vi "DRAM FIFO (U256).vi"(0 "Input Data":T5, 1 "reset":bool, 2 "Memory":T6, 3 "arbiter configuration":T4={"write grant time (clocks)"=100, "read grant time (clocks)"=100}, 5 "fifo depth":T1=8 items=["4"=2, "8"=3, "16"=4, "32"=5, "64"=6, "128"=7, "256"=8, "512"=9, "1024"=10, "2048"=11, "4096"=12, "8192"=13, "16384"=14, "32768"=15, "65536"=16, "131072"=17, "262144"=18, "524288"=19, "1048576"=20, "2097152"=21, "4194304"=22, "8388608"=23, "16777216"=24, "33554432"=25, "67108864"=26, "134217728"=27, "268435456"=28, "536870912"=29, "1073741824"=30, "2147483648"=31, "4294967296"=32], 7 "Sim_DRAM Skew":fxp<+,32,0>, 11 "input valid":bool, 14 "ready for output":bool=TRUE) -> (4 "Output Data":T5, 6 "state":T7, 8 "bank0.data":T2, 10 "Bank1.data":T2, 12 "Ready for Input":bool, 15 "Output Valid":bool)   [LabVIEW 2012, in "FIFO.lvlib"]
doc: "This VI creates a wider datapath (U256) FIFO using two DRAM U128 FIFO's (RF-RIO).\nThe outputs of the two DRAM FIFO's are cascaded to enforce writes and reads without glitches.\n\n<b> To do: </b>\nTest cascade logic for next tick glitch\nTest throughput of the DRAM"
uses:
  <userlib>/FPGA Library/Code Development/DRAM/RF-RIO/FIFO/FIFO/FPGA/FIFO.lvlib
  <userlib>/FPGA Library/Code Development/DRAM/RF-RIO/FIFO/FIFO/FPGA/Public/FIFO State.ctl
  <userlib>/FPGA Library/Code Development/DRAM/2 Bank DRAM/Data Type (256).ctl
  <userlib>/FPGA Library/Code Development/DRAM/RF-RIO/Memory/1.0.0/FPGA/Public/Timeslot Arbiter Configuration.ctl
  <userlib>/FPGA Library/Code Development/DRAM/RF-RIO/Memory/1.0.0/FPGA/Public/Retrieve Data (128-Bit).ctl
  <userlib>/FPGA Library/Code Development/DRAM/RF-RIO/Memory/1.0.0/FPGA/Public/U128.ctl
  <userlib>/FPGA Library/Code Development/DRAM/RF-RIO/FIFO/FIFO/FPGA/Private/FIFO Depth - 32-bit Address.ctl
  <userlib>/FPGA Library/Code Development/DRAM/RF-RIO/Memory/1.0.0/FPGA/Public/Write Data (128-Bit).ctl
  <instrlib>/FlexRIO/Libraries/Memory/FPGA/Interface/Read Request.ctl
  <userlib>/FPGA Library/Code Development/DRAM/2 Bank DRAM/Controls/Individual Bank Status.ctl
  <userlib>/FPGA Library/Code Development/DRAM/2 Bank DRAM/Controls/Cascaded Bank Status.ctl
  <userlib>/FPGA Library/Code Development/DRAM/RF-RIO/Memory/1.0.0/FPGA/Private/Process (DRAM 128-Bit).vi
  <instrlib>/FlexRIO/Libraries/Memory/FPGA/Memory.lvlib
  <userlib>/FPGA Library/Code Development/DRAM/RF-RIO/Memory/1.0.0/FPGA/niRFRIO Memory 1.0.0 FPGA.lvlib
panel:
  out "ready for write":bool
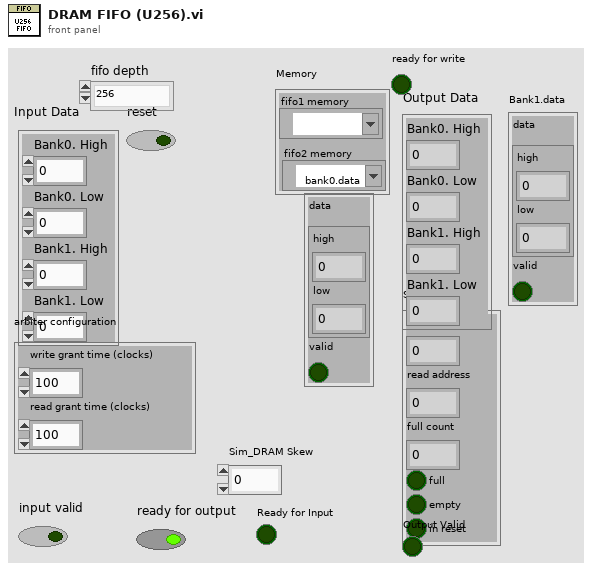
[diagram p1: front panel]
types:
  T1 = typedef "FIFO.lvlib/FIFO Depth - 32-bit Address.ctl" = u8
  T2 = typedef "FIFO.lvlib/niRFRIO Memory 1.0.0 FPGA.lvlib/Retrieve Data (128-Bit).ctl" = cluster{"data":T3, "valid":bool}
  T3 = typedef "FIFO.lvlib/niRFRIO Memory 1.0.0 FPGA.lvlib/U128.ctl" = cluster{"high":u64, "low":u64}
  T4 = typedef "FIFO.lvlib/niRFRIO Memory 1.0.0 FPGA.lvlib/Timeslot Arbiter Configuration.ctl" = cluster{"write grant time (clocks)":u16, "read grant time (clocks)":u16}
  T5 = typedef "Data Type (256).ctl" = cluster{"Bank0. High":u64, "Bank0. Low":u64, "Bank1. High":u64, "Bank1. Low":u64}
  T6 = cluster{"fifo1 memory":refnum<k21>, "fifo2 memory":refnum<k21>}
  T7 = typedef "FIFO.lvlib/FIFO State.ctl" = cluster{"write address":u32, "read address":u32, "full count":u32, "full":bool, "empty":bool, "in reset":bool}
  T8 = typedef "Cascaded Bank Status.ctl" = cluster{"Banks In Sync?":bool, "RetrieveData from Bank  0":bool, "RetrieveData from Bank  1":bool, "ready for read request":bool, "ready for write":bool}
  T9 = typedef "Individual Bank Status.ctl" = cluster{"ready for read request":bool, "ready for write":bool}
  T10 = typedef "Memory.lvlib/Read Request.ctl" = cluster{"address":u32, "valid":bool}
  T11 = typedef "FIFO.lvlib/niRFRIO Memory 1.0.0 FPGA.lvlib/Write Data (128-Bit).ctl" = cluster{"address":u32, "data":T3, "byte enables":u16, "valid":bool}
  T12 = typedef "FIFO.lvlib/FIFO State - 32-bit Address.ctl" = cluster{"write address":u32, "read address":u32, "full count":u32, "full":bool, "empty":bool}
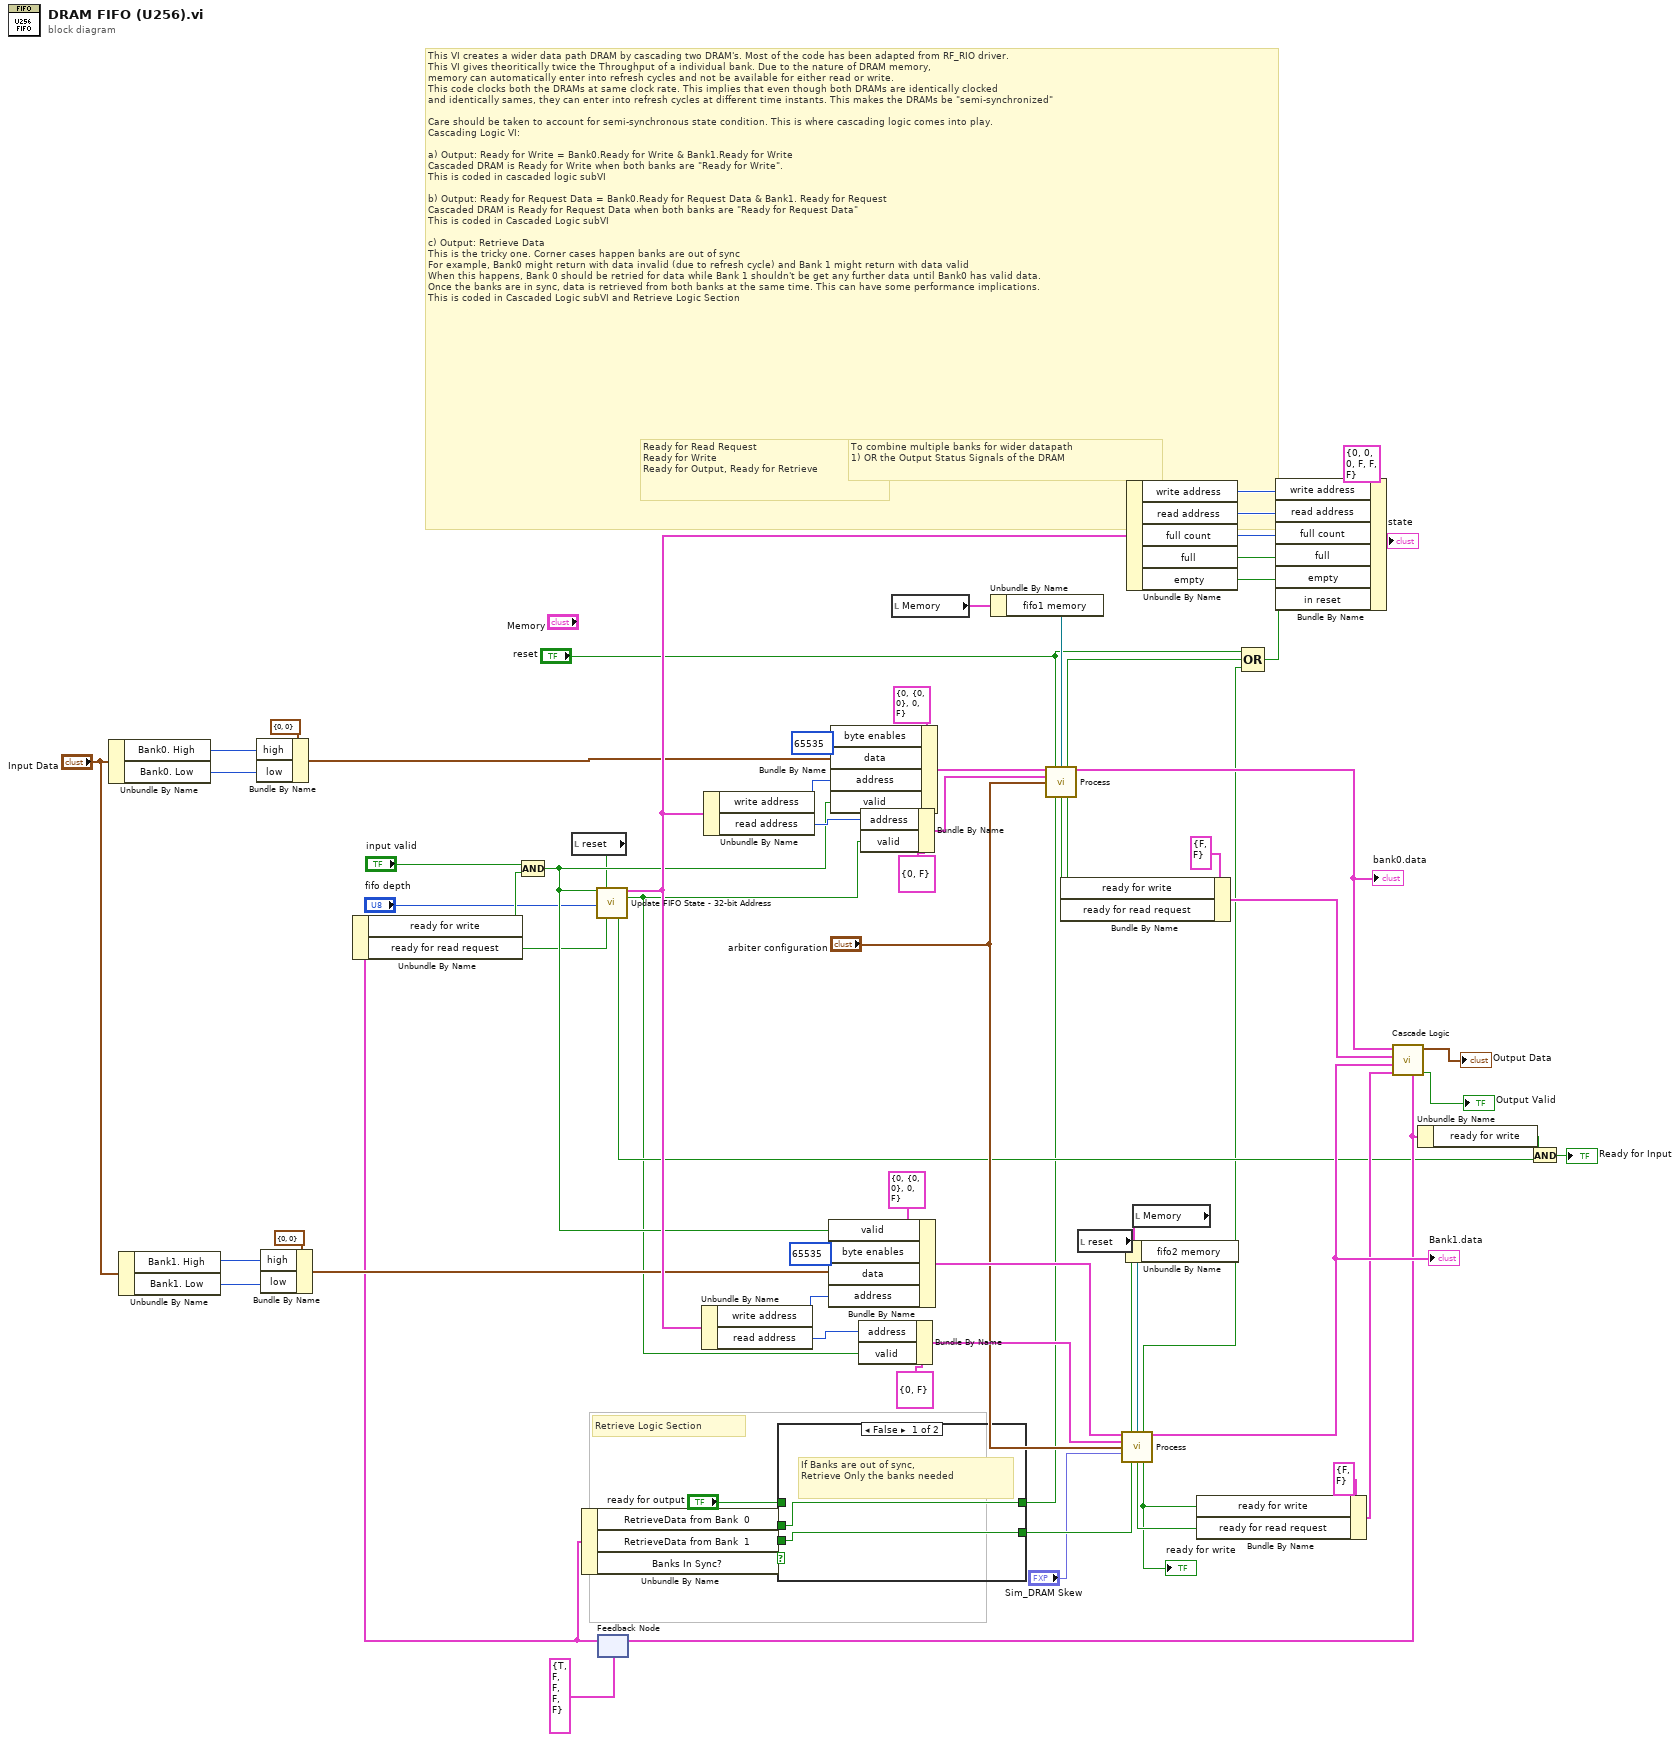
[diagram p0: block diagram]
diagram:
  # "Retrieve Logic Section"
  # "This VI creates a wider data path DRAM by cascading two DRAM's. Most of the code has been adapted from RF_RIO driver.\nThis VI gives theoritically twice the Throughput of a individual bank. Due to the nature of DRAM memory, \nmemory can automatically enter into refresh cycles and not be available for either read or write.\nThis code clocks both the DRAMs at same clock rate. This implies that even though both DRAMs are identically clocked\nand identically sames, they can enter into refresh cycles at different time instants. This makes the DRAMs be \"semi-synchronized\"\n\nCare should be taken to account for semi-synchronous state condition. This is where cascading logic comes into play.\nCascading Logic VI:\n\na) Output: Ready for Write = Bank0.Ready for Write & Bank1.Ready for Write\nCascaded DRAM is Ready for Write when both banks are \"Ready for Write\".\nThis is coded in cascaded logic subVI\n\nb) Output: Ready for Request Data = Bank0.Ready for Request Data & Bank1. Ready for Request\nCascaded DRAM is Ready for Request Data when both banks are \"Ready for Request Data\"\nThis is coded in Cascaded Logic subVI\n\nc) Output: Retrieve Data\nThis is the tricky one. Corner cases happen banks are out of sync\nFor example, Bank0 might return with data invalid (due to refresh cycle) and Bank 1 might return with data valid  \nWhen this happens, Bank 0 should be retried for data while Bank 1 shouldn't be get any further data until Bank0 has valid data.\nOnce the banks are in sync, data is retrieved from both banks at the same time. This can have some performance implications.\nThis is coded in Cascaded Logic subVI and Retrieve Logic Section"
  # "Ready for Read Request\nReady for Write\nReady for Output, Ready for Retrieve"
  # "To combine multiple banks for wider datapath\n1) OR the Output Status Signals of the DRAM"
  n1 = Unbundle By Name("Input Data") -> ("Bank0. High"=w48:u64, "Bank0. Low"=w47:u64)
  n2 = Unbundle By Name("Input Data") -> ("Bank1. High"=w43:u64, "Bank1. Low"=w42:u64)
  n3 = Bundle By Name(cluster=cluster{"high":u64, "low":u64} {"high"=0, "low"=0} ("input data"), "high"=w48, "low"=w47) -> (w46:cluster{"high":u64, "low":u64})
  n4 = Bundle By Name(cluster=cluster{"high":u64, "low":u64} {"high"=0, "low"=0} ("input data"), "high"=w43, "low"=w42) -> (w41:cluster{"high":u64, "low":u64})
  n5 = local read "reset"() -> (w17:bool)
  n6 = feedback #1(T8 {"Banks In Sync?"=TRUE, "RetrieveData from Bank  0"=FALSE, "RetrieveData from Bank  1"=FALSE, "ready for read request"=FALSE, "ready for write"=FALSE} ("Cascaded Bank Status")) -> (w21:T8)
  n7 = Unbundle By Name(w21) -> ("ready for write"=w26:bool, "ready for read request"=w1:bool)
  n8 = Compound Arithmetic op=AND("input valid", w26) -> (w33:bool)
  n9 = Unbundle By Name(w21) -> ("RetrieveData from Bank  0"=w8:bool, "RetrieveData from Bank  1"=w7:bool, "Banks In Sync?"=w22:bool)
  n10 = call <userlib>:"Update FIFO State - 32-bit Address.vi"("issue write"=w33, "reset"=w17, "fifo depth"="fifo depth", "ready for read request"=w1) -> ("state"=w52:T12, "issue read request"=w11:bool, "ready for write"=w19:bool)  [unwired: 9 in]
  n11 = Unbundle By Name(w52) -> ("write address"=w55:u32, "read address"=w57:u32)
  n12 = Unbundle By Name(w52) -> ("write address"=w70:u32, "read address"=w67:u32)
  n13 = case shown="False" w22 {
    tunnel: w8 -> [w75 _]
    tunnel: w7 -> [w74 _]
    tunnel: "ready for output" -> [_ w76]
    tunnel: [w75 w76] -> w5
    tunnel: [w74 w76] -> w4
    frame False {
      # "If Banks are out of sync,\nRetrieve Only the banks needed"
    }
    frame True {
      # "Retrieve Data = Ready for O/P"
      # "If banks are in sync, retriveve\ndata when ready for output is true"
    }
  }
  n14 = Bundle By Name(cluster=T11 {"address"=0, "data"={"high"=0, "low"=0}, "byte enables"=0, "valid"=FALSE} ("write data"), "valid"=w33, "byte enables"=u16 65535, "data"=w41, "address"=w55) -> (w51:T11)
  n15 = Bundle By Name(cluster=T11 {"address"=0, "data"={"high"=0, "low"=0}, "byte enables"=0, "valid"=FALSE} ("write data"), "byte enables"=u16 65535, "data"=w46, "address"=w70, "valid"=w33) -> (w71:T11)
  n16 = Bundle By Name(cluster=T10 {"address"=0, "valid"=FALSE} ("read request"), "address"=w57, "valid"=w11) -> (w50:T10)
  n17 = Bundle By Name(cluster=T10 {"address"=0, "valid"=FALSE} ("read request"), "address"=w67, "valid"=w11) -> (w68:T10)
  n18 = local read "Memory"() -> (w14:T6)
  n19 = Unbundle By Name(w14) -> ("fifo1 memory"=w39:refnum<k21>)
  n20 = call-poly <userlib>:"Process.vi"("write data"=w71, "reset"="reset", "memory"=w39, "read request"=w68, "arbiter configuration"="arbiter configuration", "ready for retrieve data (T)"=w5) -> ("in reset"=w58:bool, "retrieve data"=w36:T2, "ready for read request"=w28:bool, "ready for write"=w3:bool)  [unwired: 6 in]
  "bank0.data" <- w36
  n21 = Bundle By Name(cluster=T9 {"ready for read request"=FALSE, "ready for write"=FALSE} ("Bank Status Signals"), "ready for write"=w3, "ready for read request"=w28) -> (w27:T9)
  n22 = local read "reset"() -> (w16:bool)
  n23 = Unbundle By Name(w52) -> ("write address"=w64:u32, "read address"=w63:u32, "full count"=w62:u32, "full"=w61:bool, "empty"=w60:bool)
  n24 = local read "Memory"() -> (w38:T6)
  n25 = Unbundle By Name(w38) -> ("fifo2 memory"=w37:refnum<k21>)
  n26 = call-poly <userlib>:"Process.vi"("write data"=w51, "reset"=w16, "memory"=w37, "read request"=w50, "arbiter configuration"="arbiter configuration", "Sim_DRAM Skew"="Sim_DRAM Skew", "ready for retrieve data (T)"=w4) -> ("in reset"=w15:bool, "retrieve data"=w35:T2, "ready for read request"=w31:bool, "ready for write"=w9:bool)  [unwired: 5 in]
  "Bank1.data" <- w35
  "ready for write" <- w9
  n27 = Bundle By Name(cluster=T9 {"ready for read request"=FALSE, "ready for write"=FALSE} ("Bank Status Signals"), "ready for write"=w9, "ready for read request"=w31) -> (w30:T9)
  n28 = Compound Arithmetic op=OR("reset", w58, w15) -> (w40:bool)
  n29 = Bundle By Name(cluster=T7 {"write address"=0, "read address"=0, "full count"=0, "full"=FALSE, "empty"=FALSE, "in reset"=FALSE} ("state"), "write address"=w64, "read address"=w63, "full count"=w62, "full"=w61, "empty"=w60, "in reset"=w40) -> (→"state":T7)
  n30 = call <userlib>:"Cascade Logic.vi"("Bank1 Status"=w30, "Bank1 Data"=w35, "Bank0 Status"=w27, "Bank0 Data"=w36) -> ("Output Valid"=→"Output Valid":bool, "Output Data"=→"Output Data":T5, "Cascaded Bank Status"=w23:T8)  [unwired: 5 in]
  n31 = feedback-in #1(w23) -> ()
  n32 = Unbundle By Name(w23) -> ("ready for write"=w20:bool)
  n33 = And(x=w20, y=w19) -> (x .and. y?=→"Ready for Input":bool)
